vi "Test - Thermal Chamber Controller_DQMH - Update Heater State 1.vi"(8 "error in (no error)":errorcluster, 10 "Heater State Input":T1) -> (0 "error out":errorcluster, 2 "Heater State Result":T1, 3 "Success":bool)   [LabVIEW 2015]
doc: "_____\nCreated using Delacor QMH Event Scripter 4.0.0.68."
uses:
  Libraries/Thermal Chamber Controller_DQMH/Heater State--enum.ctl
  Libraries/Thermal Chamber Controller_DQMH/Thermal Chamber Controller_DQMH.lvlib
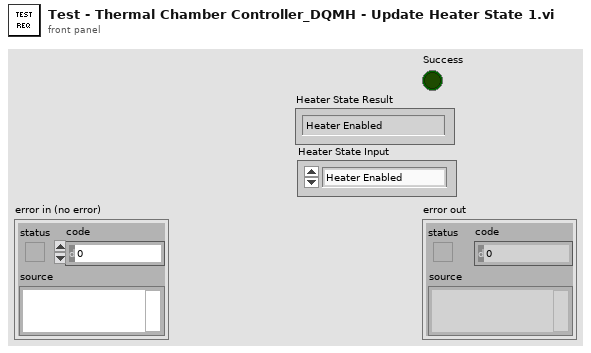
[diagram p1: front panel]
types:
  T1 = typedef "Thermal Chamber Controller_DQMH.lvlib/Heater State--enum.ctl" = enum16{"Heater Enabled", "Heater Disabled"}
  T2 = typedef "Thermal Chamber Controller_DQMH.lvlib/Broadcast Events--cluster.ctl" = cluster{"Module Did Init":refnum<user-event>, "Status Updated":refnum<user-event>, "Error Reported":refnum<user-event>, "Module Did Stop":refnum<user-event>, "Update Module Execution Status":refnum<user-event>, "Set Point Updated":refnum<user-event>, "Ramp Rate Updated":refnum<user-event>, "Heater State Updated":refnum<user-event>, "Chamber Status Updated":refnum<user-event>}
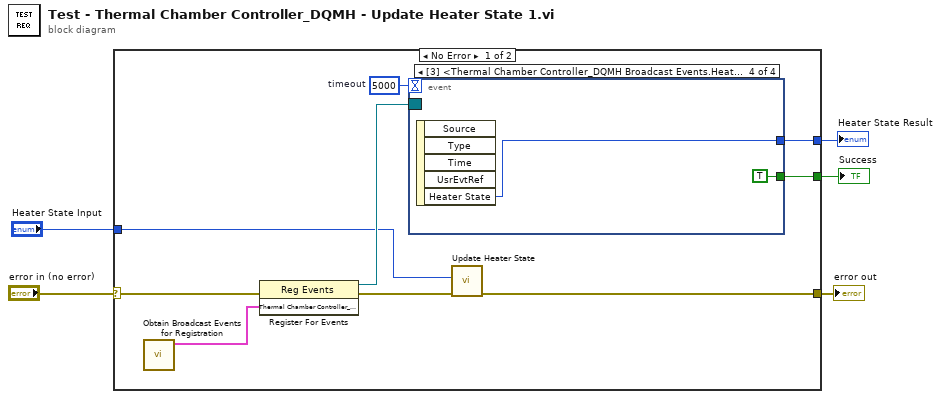
[diagram p0: block diagram]
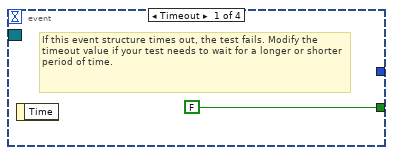
[diagram p2: hidden frame]
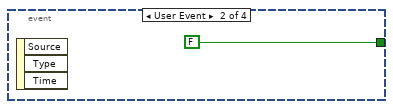
[diagram p3: hidden frame]
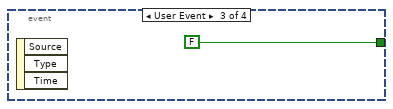
[diagram p4: hidden frame]
diagram:
  n1 = case shown="No Error" "error in (no error)" {
    selector: "error in (no error)" -> [w14 w20]
    tunnel: [w13 w20] -> w4
    tunnel: [w8 _] -> w3
    tunnel: [w7 _] -> w2
    tunnel: "Heater State Input" -> [w6 _]
    frame No Error {
      w9 = 5000  # timeout
      n2 = call "Obtain Broadcast Events for Registration.vi"() -> ("Thermal Chamber Controller_DQMH Broadcast Events"=w11:T2)  [unwired: 9 in, 2 out]
      n3 = register-events(error in=w14, w11) -> (reference out=w10:refnum<event-registration>, error out=w12:errorcluster)  [unwired: 1 in]
      n4 = event shown="[3] <Thermal Chamber Controller_DQMH Broadcast Events.Heater State Updated>: User Event" {
        selector: w10 -> [_ _ _ _]
        dyn-events: _ -> [_ _ _ _]
        timeout: w9 -> [_ _ _ _]
        tunnel: [FALSE FALSE FALSE TRUE] -> w8
        tunnel: [_ _ _ w18] -> w7
        event Timeout {
          # "If this event structure times out, the test fails. Modify the timeout value if your test needs to wait for a longer or shorter period of time."
          n5 = event-data() -> ()  [unwired: 1 in, 1 out]
        }
        event User Event {
          n6 = event-data() -> ()  [unwired: 1 in, 3 out]
        }
        event User Event {
          n7 = event-data() -> ()  [unwired: 1 in, 3 out]
        }
        event User Event {
          n8 = event-data() -> ("Heater State"=w18:T1)  [unwired: 1 in, 4 out]
        }
      }
      n9 = call "Update Heater State.vi"("error in (no error)"=w12, "Heater State"=w6) -> ("error out"=w13:errorcluster)  [unwired: 9 in]
    }
    frame Error {
    }
  }
  "error out" <- w4
  "Success" <- w3
  "Heater State Result" <- w2
